vi "Example Modbus Master - ModbusMasterWriteSingleRegisterResponseCallback Callback.vi"(4 "ModbusMasterWriteSingleRegisterResponseCallback":refnum<user-event>, 5 "Event Data":T1, 6 "Control Ref":refnum<k24>, 7 "Event Common Data":T2) -> ()   [LabVIEW 2013]
uses:
  C:/tf/play/labview/Tinkerforge.dll
  Tinkerforge.dll
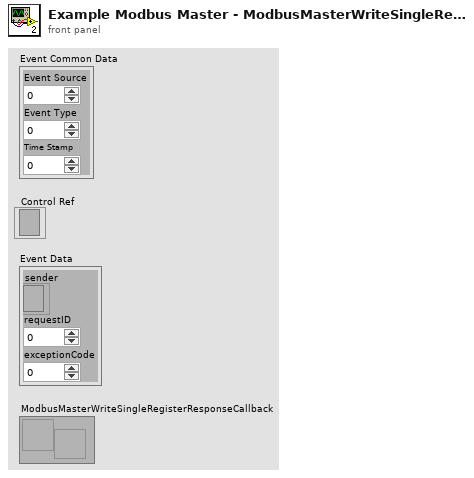
[diagram p1: front panel]
types:
  T1 = cluster{"sender":refnum<k24>, "requestID":u8, "exceptionCode":i16}
  T2 = cluster{"Event Source":i32, "Event Type":u32, "Time Stamp":u32}
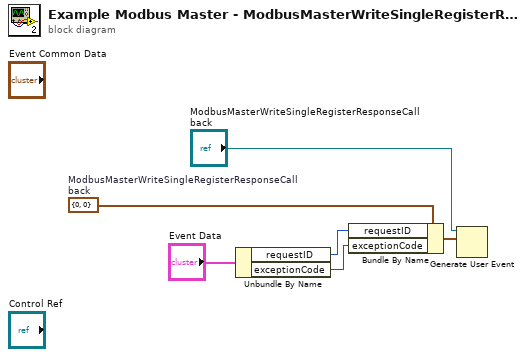
[diagram p0: block diagram]
diagram:
  w5 = cluster{"requestID":u8, "exceptionCode":i16} {"requestID"=0, "exceptionCode"=0}  # ModbusMasterWriteSingleRegisterResponseCallback
  n1 = Unbundle By Name("Event Data") -> ("requestID"=w4:u8, "exceptionCode"=w3:i16)
  n2 = Bundle By Name(cluster=w5, "requestID"=w4, "exceptionCode"=w3) -> (w2:cluster{"requestID":u8, "exceptionCode":i16})
  n3 = Generate User Event(user event="ModbusMasterWriteSingleRegisterResponseCallback", event data cluster=w2) -> ()  [unwired: 2 in, 2 out]
